vi "Read LogData.vi"(8 "error in (no error)":errorcluster, 11 "Log in":refnum<class "Log.lvclass">) -> (0 "error out":errorcluster, 2 "Log Data":T1, 3 "Log out":refnum<class "Log.lvclass">)   [LabVIEW 2017, in "Reports.lvlib" / "Log.lvclass"]
uses:
  Log.lvclass
  Log Data.ctl
  Log.lvclass/Log.ctl
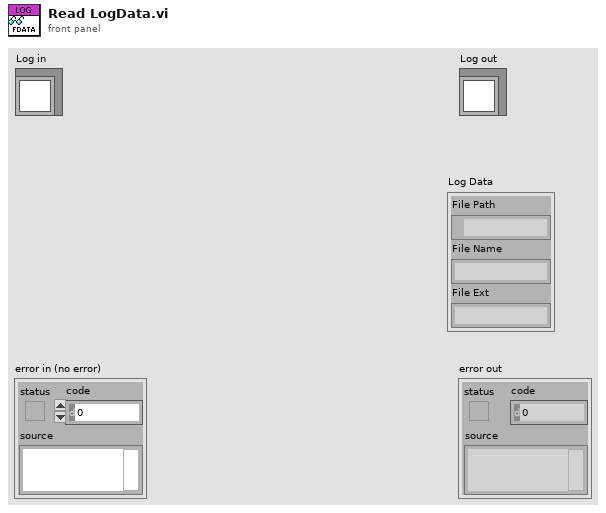
[diagram p1: front panel]
types:
  T1 = typedef "Log Data.ctl" = cluster{"File Path":path, "File Name":string, "File Ext":string}
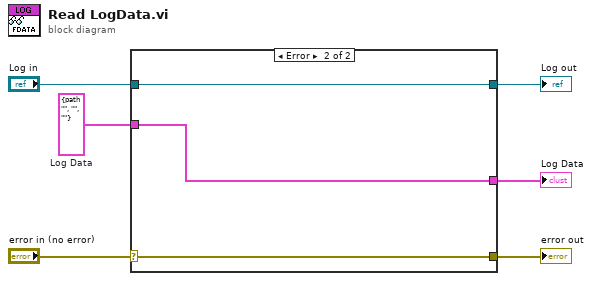
[diagram p0: block diagram]
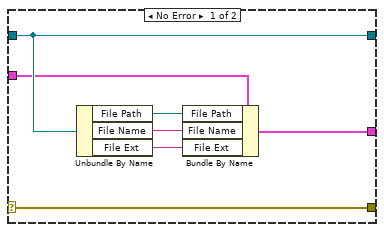
[diagram p2: hidden frame]
diagram:
  w2 = T1 {"File Path"=path "", "File Name"="", "File Ext"=""}  # Log Data
  n1 = case shown="Error" "error in (no error)" {
    selector: "error in (no error)" -> [w13 w15]
    tunnel: [w13 w15] -> w5
    tunnel: [w12 w16] -> w3
    tunnel: "Log in" -> [w12 w16]
    tunnel: w2 -> [w11 w14]
    tunnel: [w7 w14] -> w1
    frame No Error {
      n2 = Unbundle By Name(w12) -> ("File Path"=w10:path, "File Name"=w9:string, "File Ext"=w8:string)
      n3 = Bundle By Name(cluster=w11, "File Path"=w10, "File Name"=w9, "File Ext"=w8) -> (w7:T1)
    }
    frame Error {
    }
  }
  "error out" <- w5
  "Log out" <- w3
  "Log Data" <- w1
